vi "Day 9.vi"() -> ()   [LabVIEW 2023]
panel:
  out "i":i32
  in  "milliseconds to wait":u32
  out "XY Graph 2":cluster{"X":i32, "Y":i32}[](graph)
  in  "number of knots":i32=1
  out "XY Graph":cluster{"X":i32, "Y":i32}[](graph)
  out "Array":bool[][](array[boolean])
  out "Answer":i16
  in  "test":bool
  in  "test input":string="R 4\nU 4\nL 3\nD 1\nR 4\nD 1\nL 5\nR 2"
  in  "input":string="D 2\nU 1\nD 2\nR 2\nL 1\nU 2\nL 1\nU 2\nD 1\nR 1\nD 2\nR 1\nD 1\nU 2\nD 2\nR 1\nU 1\nR 1\nU 2\nR 1\nL 1\nU 2\nR 1\nL 2\nU 1\nR 1\nU 1\nR 1\nL 2\nU 2\nD 1\nU 1\nD 2\nL 1\nU 1\nL 1\nR 1\nD 1\nR 1\nD 1\nU 2\nD 1\nR 1\nU 1\nL 1\nU 2\nL 1\nD 1\nU 1\nD 1\nL 1\nU 2\nL 1\nD 2\nR 2\nL 1\nR 2\nD 1\nL 2\nD 2\nU 2\nR 1\nL 1\nD 2\nU 2\nL 1\nD 2\nU 1\nL 2\nR 2\nU 1\nD 1\nU 1\nD 1\nR 1\nD 1\nU 2\nD 1\nR 1\nD 1\nL 1\nD 1\nL 2\nU 2\nD 1\nR 1\nD 1\nL 1\nD 2\nR 2\nU 2\nD 1\nU 2\nD 1\nU 1\nL 1\nR 2\nD 2\nR 1\nD 2\nL 2\nD 2\nR 1\nL 1\nU 1\nD 2\nR 2\nU 2\nR 2\nL 1\nR 1\nL 3\nU 3\nL 3\nD 2\nU 1\nD 1\nU 2\nD 1\nR 1\nD 1\nR 2\nD 3\nU 1\nL 2\nU 1\nD 2\nR 1\nD 1\nL 2\nR 2\nU 1\nL 2\nD 2\nL 1\nU 2\nD 3\nL 1\nU 1\nR 2\nU 3\nD 1\nL 3\nU 1\nL 3\nD 1\nR 2\nL 3\nU 2\nL 2\nU 1\nL 1\nR 3\nD 3\nL 1\nR 2\nD 3\nR 2\nL 3\nD 1\nU 2\nR 3\nU 2\nR 3\nL 2\nU 1\nL 1\nD 3\nU 1\nD 1\nU 2\nD 3\nU 3\nR 1\nU 2\nL 1\nD 1\nL 2\nU 1\nD 1\nL 1\nR 3\nU 3\nL 3\nD 3\nL 2\nD 1\nU 1\nL 1\nU 3\nL 1\nD 3\nR 1\nL 1\nR 2\nU 1\nR 2\nU 3\nR 1\nD 3\nL 3\nU 2\nL 3\nR 1\nD 2\nU 3\nR 3\nD 3\nU 1\nR 3\nD 2\nR 3\nU 1\nD 1\nU 3\nR 1\nL 1\nU 2\nL 1\nU 1\nL 1\nR 1\nD 1\nR 3\nD 4\nL 2\nR 4\nU 3\nD 1\nR 4\nL 4\nR 1\nD 2\nU 3\nR 2\nD 2\nU 3\nR 4\nL 2\nD 3\nL 4\nD 4\nU 4\nR 2\nU 1\nL 3\nD 4\nU 2\nR 1\nL 3\nD 3\nR 4\nD 2\nR 2\nD 4\nU 4\nL 4\nD 4\nR 2\nD 2\nU 3\nD 3\nR 3\nL 2\nD 2\nL 2\nU 3\nL 4\nU 2\nR 4\nD 4\nL 3\nR 1\nU 1\nR 2\nL 1\nD 1\nU 2\nD 3\nL 4\nU 3\nL 1\nU 3\nR 2\nU 3\nR 1\nU 1\nR 2\nU 2\nR 1\nD 4\nU 4\nL 2\nU 2\nD 4\nU 1\nR 4\nL 4\nD 4\nU 3\nD 4\nL 4\nU 3\nL 1\nR 4\nL 3\nD 3\nU 1\nR 4\nD 3\nU 4\nL 2\nU 4\nD 3\nR 2\nD 3\nU 4\nR 4\nL 4\nR 3\nU 1\nR 4\nD 1\nL 3\nU 3\nL 3\nD 1\nL 4\nR 2\nU 1\nL 3\nR 2\nU 4\nL 1\nU 5\nR 2\nL 2\nU 2\nL 2\nR 4\nD 4\nL 5\nD 1\nR 4\nU 5\nL 1\nD 4\nU 1\nL 4\nU 3\nL 1\nR 3\nD 1\nR 2\nL 5\nU 3\nL 5\nU 4\nD 3\nL 5\nD 2\nR 4\nU 2\nL 1\nR 4\nL 5\nR 3\nL 1\nU 2\nL 4\nD 1\nR 2\nL 5\nU 3\nD 2\nR 5\nL 4\nD 2\nR 3\nD 2\nR 4\nD 3\nU 1\nD 1\nU 4\nD 2\nL 2\nR 1\nU 5\nD 5\nU 3\nR 2\nU 3\nL 5\nR 1\nU 3\nL 4\nR 2\nU 3\nD 1\nU 2\nD 2\nL 5\nR 5\nD 3\nL 1\nR 3\nU 2\nD 5\nU 1\nD 5\nR 3\nU 1\nL 5\nR 1\nD 4\nL 4\nD 1\nU 2\nL 4\nR 5\nU 5\nL 4\nD 2\nR 5\nU 1\nL 5\nD 1\nL 1\nU 5\nR 1\nL 2\nR 5\nL 5\nR 2\nL 1\nD 2\nU 1\nL 3\nR 1\nU 5\nD 1\nU 1\nL 5\nU 6\nR 6\nU 5\nD 5\nR 3\nU 1\nR 1\nL 6\nR 6\nD 5\nR 6\nD 4\nL 3\nR 6\nU 5\nD 6\nL 2\nR 1\nD 5\nR 3\nD 2\nL 1\nR 5\nU 5\nD 4\nU 3\nR 5\nU 5\nR 3\nD 5\nR 3\nU 3\nR 2\nD 5\nL 6\nD 3\nU 3\nD 6\nR 5\nU 4\nL 4\nD 3\nU 6\nL 2\nR 1\nU 4\nD 1\nL 2\nU 1\nL 3\nD 4\nU 1\nL 5\nD 1\nR 2\nU 3\nL 1\nR 1\nU 1\nL 4\nU 6\nR 6\nD 3\nU 4\nR 2\nD 5\nL 6\nD 2\nR 4\nD 2\nU 5\nD 3\nU 2\nR 6\nL 5\nR 6\nU 1\nL 5\nU 1\nL 6\nU 1\nD 4\nR 3\nD 3\nL 1\nD 3\nR 2\nL 1\nR 3\nD 4\nL 6\nU 2\nD 5\nU 3\nR 6\nU 2\nR 6\nL 5\nR 1\nU 2\nR 3\nU 1\nR 6\nL 2\nU 6\nR 5\nU 1\nR 4\nL 1\nR 3\nU 3\nL 5\nD 7\nR 2\nD 4\nR 5\nL 3\nR 6\nU 7\nL 7\nU 6\nL 2\nD 2\nR 7\nD 7\nU 3\nR 1\nU 7\nL 2\nD 3\nL 5\nR 4\nU 7\nR 3\nL 7\nD 2\nR 7\nD 5\nL 7\nD 1\nU 7\nR 5\nU 4\nD 4\nU 4\nD 4\nU 1\nR 7\nL 3\nD 3\nU 2\nL 3\nU 1\nD 7\nL 6\nR 3\nU 6\nD 1\nR 6\nD 1\nR 1\nD 7\nU 4\nR 1\nL 4\nU 3\nL 7\nR 2\nD 2\nL 6\nU 2\nR 2\nU 7\nR 5\nL 6\nR 5\nD 1\nR 4\nU 2\nL 1\nD 4\nU 5\nR 4\nD 7\nU 7\nR 1\nU 3\nR 4\nL 1\nR 6\nL 4\nU 4\nL 2\nU 3\nD 2\nL 2\nU 2\nL 6\nR 5\nD 7\nL 2\nU 5\nL 6\nR 7\nL 7\nD 2\nU 6\nD 3\nR 1\nU 1\nD 4\nL 7\nD 7\nU 5\nL 6\nD 1\nL 4\nD 1\nU 1\nL 5\nU 1\nR 5\nD 8\nR 7\nL 5\nU 3\nD 2\nR 2\nL 6\nR 1\nL 4\nR 8\nU 8\nL 5\nR 7\nD 7\nL 2\nR 5\nL 6\nD 2\nL 7\nU 3\nR 2\nD 3\nU 3\nL 6\nU 5\nD 3\nL 6\nU 5\nD 5\nL 1\nU 4\nL 8\nD 3\nL 3\nR 2\nU 6\nD 8\nU 7\nL 6\nD 2\nU 4\nD 1\nU 3\nL 6\nR 2\nD 2\nU 4\nR 8\nD 3\nR 6\nD 6\nU 1\nL 4\nU 3\nL 6\nD 8\nU 7\nD 5\nL 3\nU 4\nD 2\nR 7\nL 8\nU 1\nR 3\nD 5\nU 5\nD 6\nR 3\nL 2\nR 8\nL 3\nU 5\nL 3\nU 5\nL 7\nU 7\nL 2\nU 1\nL 5\nD 7\nU 7\nD 8\nR 2\nD 7\nU 4\nR 4\nU 6\nL 2\nU 8\nD 1\nU 1\nD 4\nL 4\nU 1\nL 5\nR 8\nU 5\nD 4\nR 2\nD 6\nL 1\nD 8\nU 4\nD 5\nL 8\nU 3\nL 5\nD 1\nU 3\nR 1\nD 7\nR 9\nU 8\nR 7\nL 3\nD 8\nU 9\nD 1\nU 7\nL 6\nU 4\nR 8\nU 1\nD 6\nR 3\nL 5\nD 3\nU 1\nL 3\nU 2\nL 3\nU 2\nR 7\nD 2\nR 7\nD 8\nR 1\nD 4\nR 1\nD 6\nR 8\nU 8\nL 2\nU 8\nL 5\nD 1\nU 7\nR 4\nL 9\nU 2\nL 3\nU 4\nL 2\nD 3\nL 4\nU 9\nD 2\nR 2\nU 9\nR 1\nL 4\nD 5\nR 9\nU 3\nL 3\nU 8\nR 5\nU 7\nD 5\nU 9\nR 3\nD 9\nR 1\nD 7\nR 3\nD 6\nL 6\nD 5\nU 9\nD 8\nU 4\nL 5\nR 6\nD 7\nR 6\nL 8\nR 3\nU 3\nR 9\nU 8\nR 6\nL 9\nU 2\nR 9\nL 8\nU 1\nR 9\nL 5\nD 5\nU 9\nL 6\nD 7\nU 3\nD 3\nR 4\nD 1\nL 4\nD 5\nL 4\nU 2\nR 9\nU 7\nL 4\nD 7\nU 9\nR 4\nD 7\nR 7\nD 4\nL 1\nD 2\nL 1\nU 7\nR 8\nD 2\nU 9\nD 6\nL 7\nR 5\nL 3\nR 5\nD 8\nL 3\nR 8\nL 6\nU 6\nL 6\nU 5\nR 7\nL 9\nU 1\nR 3\nD 7\nU 10\nD 1\nU 8\nD 8\nL 5\nU 6\nD 5\nU 9\nR 8\nD 8\nR 9\nD 2\nL 1\nD 8\nR 2\nD 6\nL 10\nR 1\nU 3\nL 8\nU 7\nR 7\nU 7\nD 6\nL 7\nU 3\nL 4\nR 9\nD 8\nU 4\nD 3\nL 8\nR 7\nU 1\nL 9\nD 10\nU 2\nL 5\nU 3\nL 4\nR 10\nL 2\nD 6\nL 6\nD 2\nU 5\nD 3\nR 9\nD 2\nU 1\nD 5\nU 9\nD 7\nR 2\nU 5\nR 4\nD 9\nU 6\nL 10\nD 3\nU 1\nL 1\nD 9\nU 2\nL 8\nU 3\nR 5\nU 7\nD 8\nR 5\nL 8\nU 9\nL 1\nD 5\nU 8\nR 4\nD 7\nU 4\nR 10\nU 9\nR 9\nU 7\nR 3\nU 10\nR 5\nU 7\nR 6\nU 10\nR 9\nU 8\nD 8\nL 1\nU 2\nD 1\nR 9\nU 10\nD 6\nL 3\nD 4\nR 11\nD 11\nR 7\nU 3\nL 3\nU 11\nD 11\nU 5\nR 9\nU 3\nR 4\nD 1\nU 11\nR 2\nL 7\nR 8\nL 2\nD 4\nU 4\nL 9\nR 10\nL 3\nR 7\nD 7\nL 9\nU 6\nL 5\nD 8\nU 4\nD 4\nL 4\nD 2\nU 8\nR 4\nD 4\nU 10\nD 5\nR 5\nD 5\nU 8\nD 2\nL 6\nU 8\nL 2\nD 8\nR 5\nD 5\nU 1\nD 1\nL 9\nR 7\nU 2\nL 7\nR 1\nL 1\nU 2\nR 10\nD 2\nU 8\nL 1\nR 6\nL 3\nR 4\nD 6\nL 2\nD 11\nR 8\nD 11\nL 3\nR 4\nL 10\nU 7\nL 9\nU 4\nL 8\nD 6\nU 8\nR 7\nL 5\nR 8\nL 4\nU 6\nR 5\nU 7\nD 3\nL 8\nU 2\nR 7\nD 3\nR 4\nD 11\nL 8\nU 6\nD 1\nR 11\nL 7\nD 4\nR 4\nL 4\nU 5\nL 8\nR 7\nU 8\nD 12\nR 9\nD 8\nR 7\nL 9\nR 2\nD 1\nL 7\nD 3\nL 1\nR 5\nU 1\nD 12\nR 4\nU 1\nD 4\nL 9\nU 10\nR 5\nD 11\nR 2\nL 3\nU 8\nR 5\nD 8\nU 12\nD 6\nR 2\nD 5\nR 12\nU 7\nL 2\nU 4\nD 5\nU 8\nR 12\nU 1\nL 11\nU 7\nD 10\nL 6\nD 6\nR 1\nL 6\nD 2\nU 5\nR 6\nD 8\nR 4\nL 7\nD 2\nL 7\nD 8\nU 10\nR 1\nU 6\nR 5\nL 4\nR 8\nD 9\nR 5\nU 11\nD 4\nU 11\nR 8\nL 8\nU 2\nR 11\nL 12\nU 7\nL 12\nU 10\nR 3\nD 11\nR 1\nL 8\nD 2\nL 5\nR 4\nU 3\nD 9\nR 8\nD 11\nL 12\nR 11\nL 4\nR 10\nD 6\nU 4\nR 6\nD 6\nU 9\nR 12\nU 5\nR 8\nL 10\nD 1\nU 7\nD 12\nL 3\nU 10\nD 2\nU 6\nD 12\nR 3\nU 2\nD 2\nU 3\nD 11\nR 2\nU 2\nD 9\nR 11\nD 4\nU 6\nR 11\nL 9\nR 10\nD 13\nL 2\nD 2\nL 4\nD 13\nR 7\nL 3\nU 8\nD 5\nR 7\nD 7\nU 13\nD 5\nU 5\nL 12\nD 9\nL 2\nD 6\nU 13\nR 2\nD 10\nL 9\nD 7\nR 2\nU 3\nD 2\nL 3\nR 9\nU 3\nL 12\nU 4\nR 1\nU 13\nR 4\nU 1\nD 10\nR 10\nD 10\nU 5\nL 7\nD 8\nR 1\nD 12\nL 13\nR 10\nD 6\nR 9\nU 4\nR 9\nU 1\nL 3\nR 3\nD 8\nU 6\nL 11\nR 8\nD 5\nU 2\nL 9\nR 7\nL 7\nD 8\nL 12\nR 12\nU 9\nD 9\nU 7\nD 10\nL 3\nR 3\nD 8\nL 11\nU 8\nD 7\nU 11\nL 4\nD 4\nR 3\nU 4\nR 6\nD 5\nU 5\nL 8\nU 4\nL 9\nU 6\nL 8\nD 3\nU 12\nD 5\nL 8\nD 11\nU 4\nR 12\nU 7\nL 5\nD 4\nR 4\nU 7\nR 9\nL 5\nU 2\nL 3\nD 2\nR 6\nU 2\nR 8\nD 10\nU 14\nL 3\nR 4\nU 10\nR 7\nL 11\nR 7\nU 4\nR 8\nL 14\nD 11\nU 12\nR 10\nL 8\nR 11\nL 4\nU 1\nL 2\nR 7\nU 13\nD 5\nU 2\nL 6\nD 7\nR 5\nU 4\nD 10\nU 5\nD 2\nR 9\nU 13\nL 10\nU 1\nR 10\nD 14\nL 5\nR 12\nL 7\nD 2\nL 2\nD 5\nR 4\nU 6\nD 7\nR 12\nU 9\nD 9\nR 6\nU 1\nD 14\nU 14\nD 14\nL 7\nR 10\nU 3\nD 2\nR 10\nL 14\nR 7\nD 5\nU 1\nL 8\nU 2\nD 3\nU 6\nL 11\nR 13\nL 10\nD 9\nU 5\nR 6\nU 2\nD 7\nU 5\nL 6\nR 8\nD 11\nR 14\nD 5\nR 10\nL 13\nR 1\nU 4\nL 9\nR 2\nD 1\nU 10\nD 6\nU 3\nR 13\nL 9\nR 2\nD 3\nR 14\nL 2\nR 14\nU 1\nR 7\nL 1\nU 6\nD 6\nR 10\nL 12\nD 10\nR 11\nD 13\nL 3\nR 2\nL 1\nR 10\nU 1\nL 7\nR 5\nD 6\nU 11\nL 8\nR 7\nD 10\nU 13\nR 12\nD 8\nL 7\nU 8\nR 14\nU 10\nL 6\nD 15\nR 8\nL 10\nU 13\nL 3\nU 13\nL 9\nR 4\nD 6\nR 12\nL 12\nR 4\nU 12\nD 6\nR 2\nL 11\nR 7\nD 1\nU 4\nR 14\nU 6\nD 1\nU 15\nD 14\nR 3\nD 14\nL 1\nR 9\nL 2\nD 11\nR 11\nD 10\nR 1\nL 9\nU 6\nR 8\nL 4\nR 9\nU 13\nD 15\nL 2\nD 2\nL 2\nD 6\nR 10\nU 10\nL 8\nD 11\nL 8\nR 10\nU 3\nR 7\nU 15\nR 11\nL 10\nU 2\nR 8\nL 8\nD 5\nR 11\nU 7\nL 13\nD 15\nU 4\nD 10\nR 11\nD 6\nL 2\nU 3\nR 2\nL 1\nD 14\nU 5\nL 14\nD 13\nR 12\nU 8\nR 1\nL 14\nU 6\nD 10\nR 3\nU 8\nL 2\nR 6\nD 10\nU 9\nL 2\nD 13\nL 13\nD 9\nL 10\nU 14\nR 11\nL 14\nU 10\nL 6\nD 14\nL 11\nR 4\nL 9\nU 3\nD 13\nL 5\nR 16\nU 3\nL 9\nD 6\nR 15\nU 6\nL 4\nR 10\nD 12\nR 4\nD 2\nU 11\nD 13\nR 6\nU 15\nR 14\nD 14\nU 8\nR 9\nL 5\nD 16\nU 9\nR 15\nD 13\nR 3\nL 2\nR 3\nU 14\nD 9\nU 2\nD 6\nU 9\nD 7\nL 13\nD 7\nL 5\nR 3\nU 2\nL 13\nR 9\nD 1\nL 16\nD 8\nR 12\nU 15\nR 4\nD 15\nL 12\nD 13\nR 4\nL 2\nU 5\nR 13\nL 15\nD 12\nL 3\nD 13\nL 5\nD 16\nL 11\nD 13\nU 1\nD 9\nL 10\nU 11\nD 12\nU 11\nD 14\nU 16\nD 14\nU 10\nR 7\nL 11\nR 14\nU 11\nR 5\nU 1\nD 16\nR 16\nL 9\nU 7\nD 7\nR 8\nD 7\nU 10\nL 7\nD 6\nU 4\nD 2\nL 3\nD 3\nL 2\nR 3\nL 9\nD 2\nR 12\nD 11\nU 11\nL 14\nU 4\nL 12\nR 13\nL 9\nD 11\nR 12\nL 15\nR 15\nL 15\nR 16\nU 17\nD 4\nL 9\nU 9\nD 17\nL 8\nU 15\nD 17\nU 9\nR 4\nU 6\nL 1\nD 7\nR 3\nD 11\nL 10\nR 1\nU 14\nD 13\nR 7\nL 8\nU 16\nL 16\nU 12\nD 3\nR 4\nD 8\nR 8\nD 1\nL 12\nR 16\nD 3\nR 7\nD 16\nU 11\nR 6\nD 13\nR 4\nL 3\nR 6\nU 1\nR 4\nD 4\nU 13\nL 7\nD 17\nR 4\nD 6\nL 1\nU 17\nL 16\nU 12\nL 11\nR 1\nL 11\nD 8\nU 15\nD 6\nL 5\nU 16\nR 6\nD 11\nL 17\nD 7\nL 1\nD 8\nL 16\nU 8\nR 4\nL 17\nD 2\nL 1\nU 16\nD 8\nL 17\nU 12\nD 4\nR 1\nD 12\nU 2\nL 11\nU 17\nL 3\nR 7\nL 10\nU 16\nR 8\nU 6\nL 3\nD 15\nL 11\nR 7\nU 14\nR 8\nL 9\nD 6\nL 3\nU 17\nR 1\nD 13\nU 15\nL 18\nU 11\nR 3\nU 16\nD 12\nR 1\nD 6\nL 17\nR 9\nL 6\nU 2\nD 2\nU 16\nD 12\nR 1\nU 17\nR 16\nD 12\nU 3\nD 11\nL 13\nU 11\nR 15\nU 13\nD 11\nU 8\nL 3\nD 1\nL 7\nR 9\nD 18\nR 17\nU 2\nL 16\nD 8\nL 14\nD 11\nR 4\nD 12\nU 5\nD 6\nU 2\nD 4\nL 1\nR 11\nD 3\nU 10\nL 1\nR 16\nU 10\nL 17\nD 5\nR 16\nU 18\nR 1\nD 16\nR 14\nD 11\nU 13\nD 13\nR 5\nL 9\nU 11\nR 18\nL 14\nU 14\nL 18\nR 15\nD 10\nU 10\nR 17\nU 12\nL 2\nD 11\nR 15\nU 3\nR 17\nL 1\nR 1\nU 1\nL 8\nU 15\nR 15\nL 12\nU 2\nR 1\nL 9\nR 3\nL 6\nR 18\nD 9\nR 12\nU 6\nL 17\nR 11\nD 8\nR 17\nD 12\nL 2\nR 9\nU 4\nD 17\nR 18\nD 12\nL 9\nR 16\nU 5\nR 1\nL 12\nR 9\nL 8\nU 8\nR 2\nU 9\nL 2\nD 18\nU 11\nL 17\nU 3\nL 11\nR 3\nL 5\nD 1\nR 4\nU 10\nD 18\nR 10\nD 10\nL 5\nR 7\nD 2\nR 2\nL 18\nU 4\nD 10\nU 16\nD 1\nL 2\nU 17\nD 5\nU 9\nR 13\nD 6\nR 14\nD 10\nL 15\nR 13\nL 6\nU 11\nR 6\nL 4\nR 19\nL 4\nD 13\nR 1\nL 9\nD 4\nR 12\nU 18\nD 3\nU 17\nR 19\nL 6\nR 6\nD 8\nR 12\nL 10\nR 3\nU 5\nL 2\nD 7\nL 9\nD 16\nL 16\nU 14\nL 12\nR 2\nL 17\nR 18\nD 12\nR 16\nD 19\nU 6\nD 19\nU 13\nR 4\nD 18\nL 14\nU 14\nD 12\nR 10\nL 13\nD 10\nU 10\nD 2\nU 18\nL 19\nR 15\nD 6\nL 1\nD 10\nR 7\nD 2\nR 19\nD 5\nU 19\nL 13\nU 17\nL 3\nR 19\nU 9\nL 7\nD 6\nR 12\nL 10\nR 9\nD 9\nU 13\nR 7\nL 1\nU 1\nD 17\n"
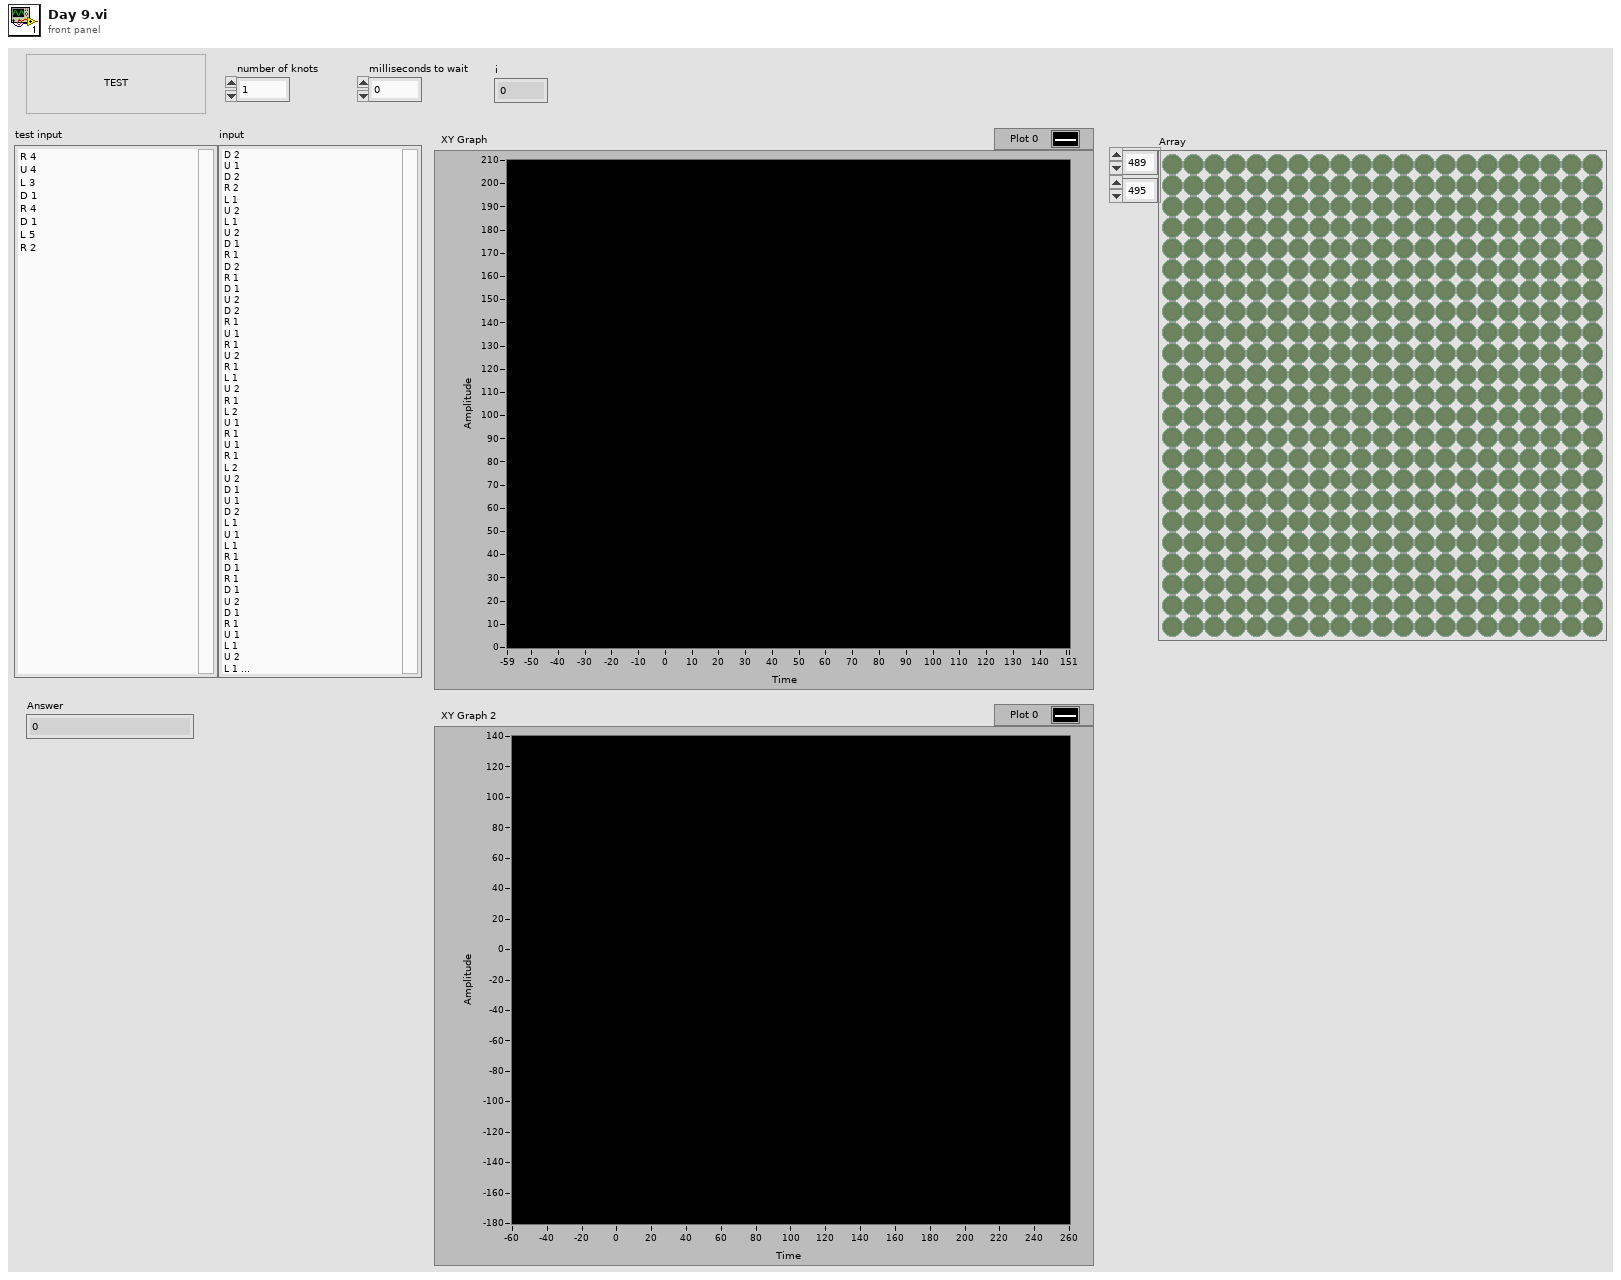
[diagram p1: front panel]
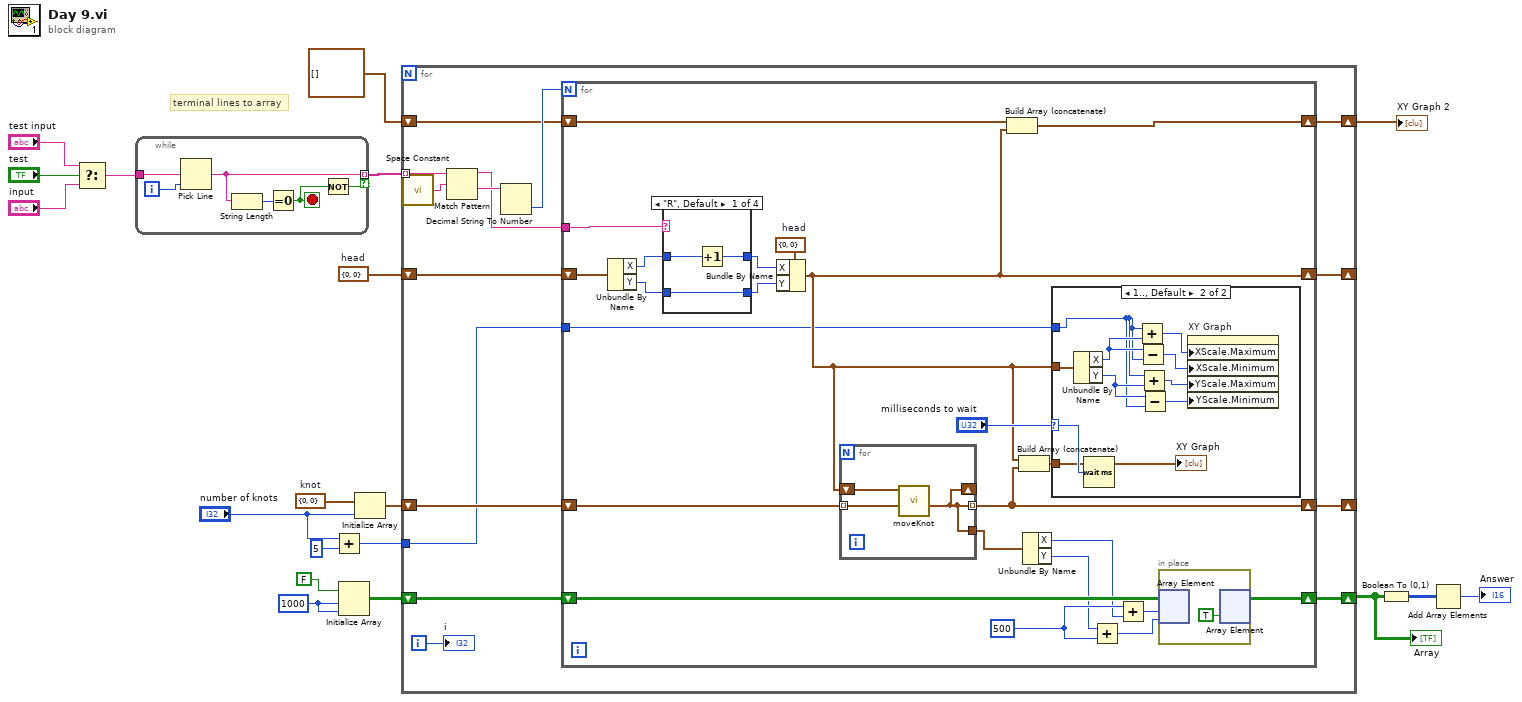
[diagram p0: block diagram]
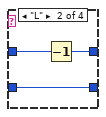
[diagram p3: hidden frame]
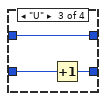
[diagram p4: hidden frame]
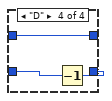
[diagram p5: hidden frame]
diagram:
  w10 = cluster{"X":i32, "Y":i32} {"X"=0, "Y"=0}  # head
  w9 = cluster{"X":i32, "Y":i32} {"X"=0, "Y"=0}  # knot
  w13 = 1000 ("dimension size")
  # "terminal lines to array"
  n1 = Select(t="test input", s="test", f="input") -> (s? t:f=w18:string)
  n2 = while {
    tunnel: w18 -> [w23]
    tunnel: [w22] -> w15 mode=indexing if=w20
    i -> [w24]
    stop <- w21 stop-if-true
    n3 = Pick Line(multi-line string=w23, line index=w24) -> (output string=w22:string)  [unwired: 1 in]
    n4 = String Length(string=w22) -> (length=w25:i32)
    n5 = Equal To 0?(x=w25) -> (x = 0?=w21:bool)
    n6 = Not(x=w21) -> (.not. x?=w20:bool)
  }
  n7 = Add(x="number of knots", y=5) -> (x+y=w2:i32)
  n8 = Initialize Array(FALSE, w13, w13) -> (w12:bool[][])
  n9 = Initialize Array(w9, "number of knots") -> (w8:cluster{"X":i32, "Y":i32}[])
  n10 = for {
    tunnel: w15 -> [w40] mode=indexing
    shift-right: [w35] -> _
    shift-left: w10 -> [w34]
    shift-right: [w32] -> w6
    shift-left: w12 -> [w33]
    shift-right: [w30] -> _
    shift-left: w8 -> [w31]
    shift-right: [w29] -> w4
    shift-left: cluster{"X":i32, "Y":i32}[] [] -> [w28]
    tunnel: w2 -> [w26]
    i -> [w27]
    n11 = call <vilib>:"Space Constant.vi"() -> ("String"=w39:string)
    n12 = Match Pattern(string=w40, regular expression=w39) -> (before substring=w37:string, after substring=w38:string)  [unwired: 1 in, 2 out]
    n13 = Decimal String To Number(string=w38) -> (number=w36:i32)  [unwired: 2 in, 1 out]
    n14 = for {
      N: w36 -> [_]
      tunnel: w37 -> [w52]
      shift-right: [w42] -> w35
      shift-left: w34 -> [w51]
      shift-right: [w62] -> w32
      shift-left: w33 -> [w63]
      shift-right: [w45] -> w30
      shift-left: w31 -> [w56]
      shift-right: [w46] -> w29
      shift-left: w28 -> [w47]
      tunnel: w26 -> [w41]
      w55 = cluster{"X":i32, "Y":i32} {"X"=0, "Y"=0}  # head
      w59 = 500 ("y")
      n15 = Unbundle By Name(w51) -> ("X"=w49:i32, "Y"=w50:i32)
      n16 = case shown="\"R\", Default" w52 {
        tunnel: w49 -> [w79 w82 w84 w88]
        tunnel: [w78 w81 w84 w88] -> w54
        tunnel: [w77 w80 w83 w86] -> w53
        tunnel: w50 -> [w77 w80 w85 w87]
        frame "R", Default {
          n17 = Increment(x=w79) -> (x+1=w78:i32)
        }
        frame "L" {
          n18 = Decrement(x=w82) -> (x-1=w81:i32)
        }
        frame "U" {
          n19 = Increment(x=w85) -> (x+1=w83:i32)
        }
        frame "D" {
          n20 = Decrement(x=w87) -> (x-1=w86:i32)
        }
      }
      n21 = Bundle By Name(cluster=w55, "X"=w54, "Y"=w53) -> (w42:cluster{"X":i32, "Y":i32})
      n22 = for {
        tunnel: w56 -> [w76] mode=indexing
        tunnel: [w74] -> w45 mode=indexing
        tunnel: [w74] -> w48
        shift-right: [w74] -> _
        shift-left: w42 -> [w75]
        n23 = call "moveKnot.vi"("knot"=w76, "head"=w75) -> ("knot"=w74:cluster{"X":i32, "Y":i32})  [unwired: 9 in]
      }
      n24 = Build Array (concatenate)(w47, w42) -> (w46:cluster{"X":i32, "Y":i32}[])
      n25 = Build Array (concatenate)(w42, w45) -> (w43:cluster{"X":i32, "Y":i32}[])
      n26 = Unbundle By Name(w48) -> ("X"=w57:i32, "Y"=w58:i32)
      n27 = case shown="1.., Default" "milliseconds to wait" {
        selector: "milliseconds to wait" -> [_ w73]
        tunnel: w43 -> [_ w72]
        tunnel: w42 -> [_ w65]
        tunnel: w41 -> [_ w64]
        frame 0 {
        }
        frame 1.., Default {
          n28 = Unbundle By Name(w65) -> ("X"=w67:i32, "Y"=w71:i32)
          n29 = Wait (ms)(milliseconds to wait=w73) -> ()  [unwired: 1 out]
          n30 = Add(x=w64, y=w67) -> (x+y=w66:i32)
          n31 = Subtract(x=w67, y=w64) -> (x-y=w68:i32)
          n32 = Add(x=w64, y=w71) -> (x+y=w69:i32)
          n33 = Subtract(x=w71, y=w64) -> (x-y=w70:i32)
          n34 = property on="XY Graph" class="XYGraph (strict)"("XScale.Maximum"=w66, "XScale.Minimum"=w68, "YScale.Maximum"=w69, "YScale.Minimum"=w70) -> ()  [unwired: 2 in, 2 out]
          "XY Graph" <- w72
        }
      }
      n35 = Add(x=w58, y=w59) -> (x+y=w60:i32)
      n36 = Add(x=w59, y=w57) -> (x+y=w61:i32)
      n37 = in-place {
        n38 = in-place-array #1(w63, w61, w60) -> ()  [unwired: 1 out]
        n39 = in-place-array #1(TRUE ("element")) -> (w62:bool[][])  [unwired: 2 out]
      }
    }
    "i" <- w27
  }
  "Array" <- w6
  "XY Graph 2" <- w4
  n40 = Boolean To (0,1)(Boolean=w6) -> (0, 1=w7:i16[][])
  n41 = Add Array Elements(numeric array=w7) -> (sum=→"Answer":i16)
